vi "Write userName.vi"(8 "error in (no error)":errorcluster, 10 "userName":string, 11 "FTP in":refnum<class "FTP.lvclass">) -> (0 "error out":errorcluster, 3 "FTP out":refnum<class "FTP.lvclass">)   [LabVIEW 2017, in "FTP_UpgradeCSMF.lvlib" / "FTP.lvclass"]
uses:
  FTP.lvclass
  FTP.lvclass/FTP.ctl
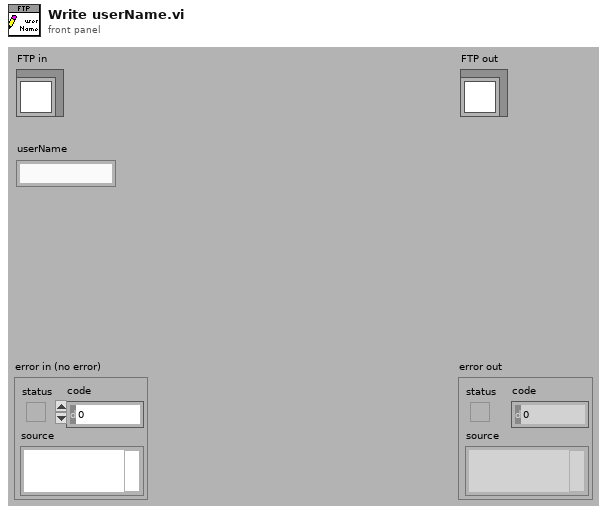
[diagram p1: front panel]
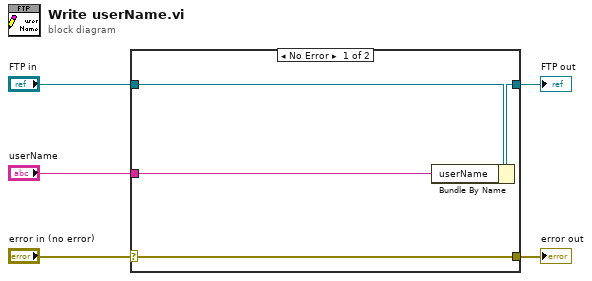
[diagram p0: block diagram]
diagram:
  n1 = case shown="No Error" "error in (no error)" {
    selector: "error in (no error)" -> [w9 w10]
    tunnel: [w9 w10] -> w4
    tunnel: [w7 w11] -> w2
    tunnel: "FTP in" -> [w8 w11]
    tunnel: "userName" -> [w6 _]
    frame No Error {
      n2 = Bundle By Name(cluster=w8, "userName"=w6) -> (w7:refnum<class "FTP.lvclass">)
    }
    frame Error {
    }
  }
  "error out" <- w4
  "FTP out" <- w2
